vi "Set Name.vi"(8 "error in (no error)":errorcluster, 10 "Name":string, 11 "Type in":variant) -> (0 "error out":errorcluster, 3 "Type out":variant)   [LabVIEW 2015, in "Scripting.lvlib"]
uses:
  Scripting.lvlib
  <vilib>/Utility/Data Type/NI_Data Type.lvlib
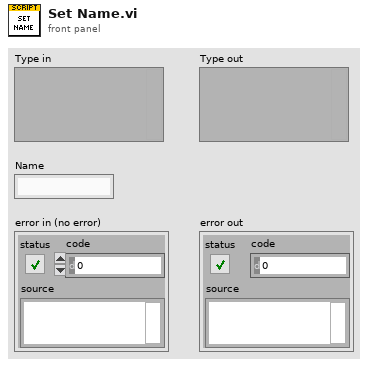
[diagram p1: front panel]
types:
  T1 = typedef "NI_Data Type.lvlib/Type Definition Info.ctl" = cluster{"Name":string, "Timestamp":u32}
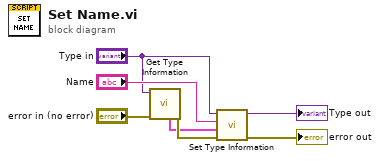
[diagram p0: block diagram]
diagram:
  n1 = call <vilib>:"Get Type Information.vi"("error in (no error)"="error in (no error)", "Variant"="Type in") -> ("error out"=w5:errorcluster, "Type Definition Info"=w4:T1)  [unwired: 5 in, 3 out]
  n2 = call <vilib>:"Set Type Information.vi"("error in (no error)"=w5, "Type Definition Info"=w4, "Name"="Name", "Variant in"="Type in") -> ("error out"=→"error out":errorcluster, "Variant out"=→"Type out":variant)  [unwired: 6 in]
